vi "micToWav.vi"(5 "filename":path=path "\\\\nas.ls.berkeley.edu\\111lab/Student-Redirect$/aguilar/My Documents/Final Sounds/loopGain.wav", 6 "Sample Length (s)":i32=5, 7 "dt":dbl=0.0001) -> (4 "error out":errorcluster)   [LabVIEW 2012]
panel:
  out "Numeric":i32
  out "Waveform Graph 3":waveform(dbl)[](graph)
  out "Waveform Graph":dbl[](graph)
  out "Waveform Graph 2":dbl[](graph)
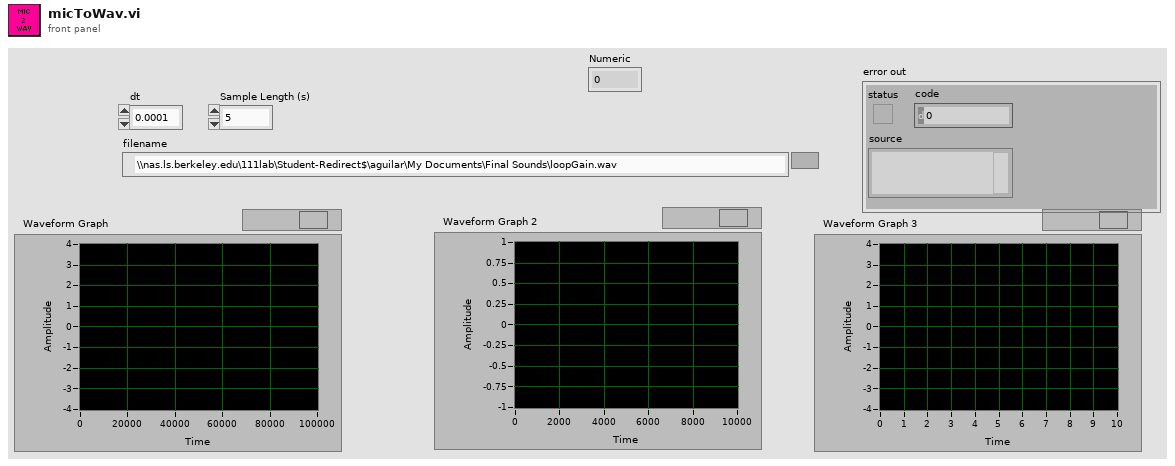
[diagram p1: front panel]
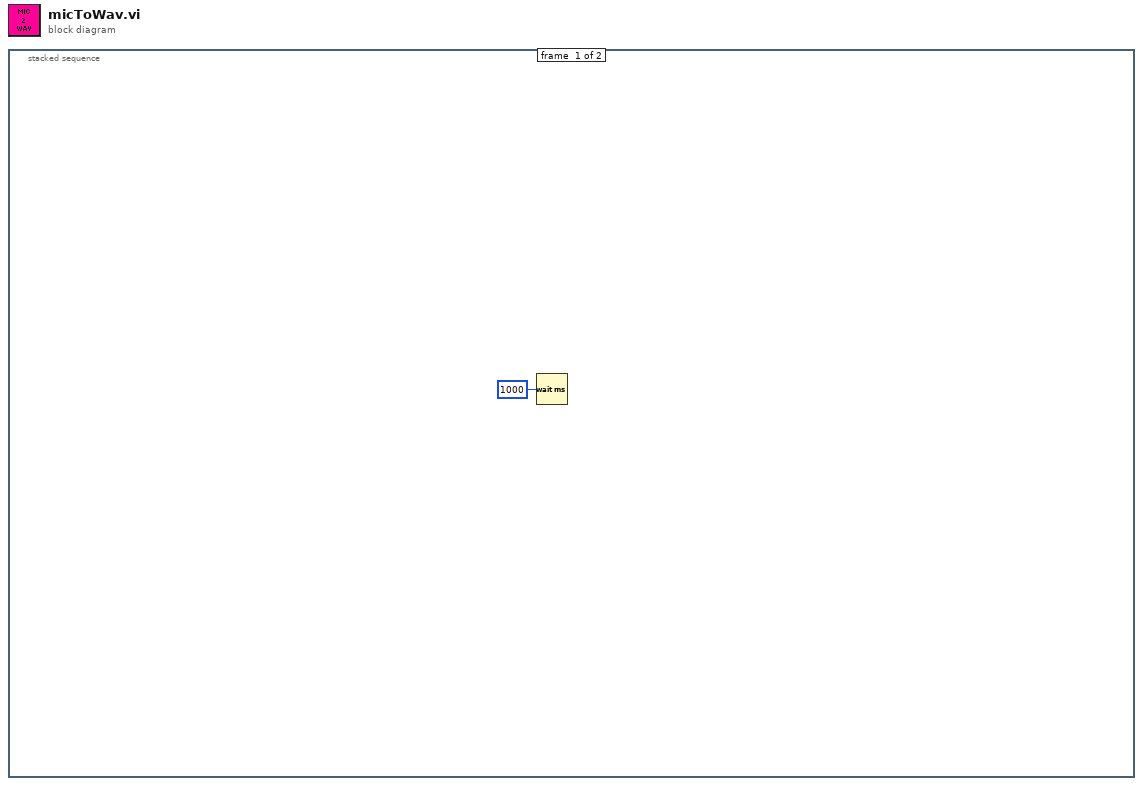
[diagram p0: block diagram]
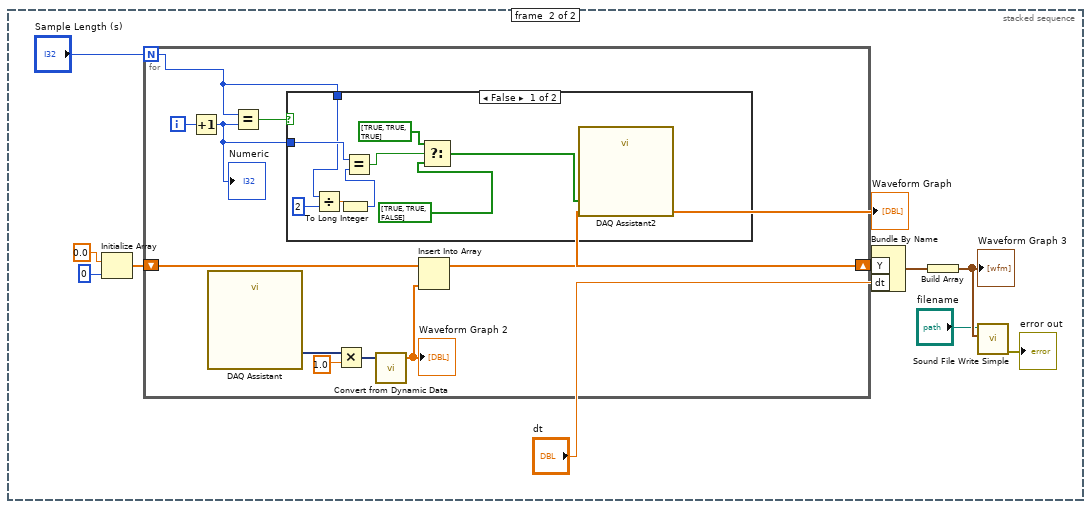
[diagram p2: hidden frame]
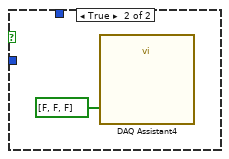
[diagram p3: hidden frame]
diagram:
  n1 = stacked-sequence {
    frame #0 {
      n2 = Wait (ms)(milliseconds to wait=u32 1000) -> ()  [unwired: 1 out]
    }
    frame #1 {
      n3 = Initialize Array(0.0 ("element"), 0 ("dimension size")) -> (w10:dbl[])
      n4 = for {
        N: "Sample Length (s)" -> [w12]
        shift-right: [w21] -> w6
        shift-left: w10 -> [w19]
        i -> [w14]
        n5 = Increment(x=w14) -> (x+1=w13:i32)
        "Numeric" <- w13
        n6 = call "DAQ Assistant"() -> ("data"=w18:dynamicdata)  [unwired: 17 in, 2 out]
        n7 = Equal?(x=w12, y=w13) -> (x = y?=w15:bool)
        n8 = case shown="False" w15 {
          tunnel: w13 -> [w30 _]
          tunnel: w12 -> [w29 _]
          frame False {
            n9 = Divide(x=w29, y=2) -> (x/y=w25:dbl)
            n10 = To Long Integer(number=w25) -> (32bit integer=w24:i32)
            n11 = Equal?(x=w30, y=w24) -> (x = y?=w27:bool)
            n12 = Select(t=bool[] [TRUE, TRUE, TRUE] ("data"), s=w27, f=bool[] [TRUE, TRUE, FALSE] ("data")) -> (s? t:f=w22:bool[])
            n13 = call "DAQ Assistant2"("data"=w22) -> ()  [unwired: 17 in, 2 out]
          }
          frame True {
            n14 = call "DAQ Assistant4"("data"=bool[] [FALSE, FALSE, FALSE]) -> ()  [unwired: 17 in, 2 out]
          }
        }
        n15 = Multiply(x=w18, y=1.0) -> (x*y=w17:dynamicdata)
        n16 = call "Convert from Dynamic Data"("Dynamic Data Type"=w17) -> ("Array"=w20:dbl[])  [unwired: 3 in]
        "Waveform Graph 2" <- w20
        n17 = Insert Into Array(array=w19, new element=w20) -> (w21:dbl[])  [unwired: 1 in]
      }
      "Waveform Graph" <- w6
      n18 = Bundle By Name("Y"=w6, "dt"="dt") -> (w5:waveform(dbl))  [unwired: 1 in]
      n19 = Build Array(w5) -> (w4:waveform(dbl)[])
      "Waveform Graph 3" <- w4
      n20 = call <vilib>:"Sound File Write Simple.vi"("data"=w4, "path"="filename") -> ("error out"=→"error out":errorcluster)  [unwired: 8 in, 1 out]
    }
  }
